vi "Read FOAD.vi"(8 "error in (no error)":errorcluster, 11 "Detector Manager in":refnum<class "Detector Manager.lvclass">=refnum) -> (0 "error out":errorcluster, 2 "Father Of All Detectors.lvclass":refnum<class "Father Of All Detectors.lvclass">, 3 "Detector Manager out":refnum<class "Detector Manager.lvclass">)   [LabVIEW 2026, in "TALOS.lvlib" / "Detector Manager.lvlib" / "Detector Manager.lvclass"]
uses:
  Detector Manager.lvclass
  Classes/Father of all Detectors/Father Of All Detectors.lvclass
  Detector Manager.lvclass/Detector Manager.ctl
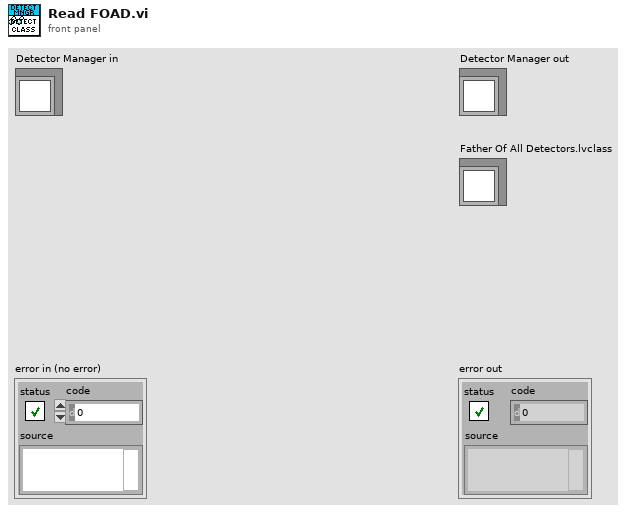
[diagram p1: front panel]
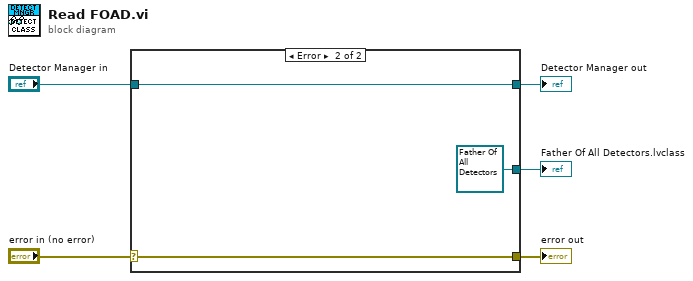
[diagram p0: block diagram]
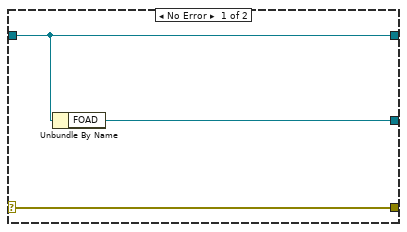
[diagram p2: hidden frame]
diagram:
  n1 = case shown="Error" "error in (no error)" {
    selector: "error in (no error)" -> [w8 w10]
    tunnel: [w8 w10] -> w4
    tunnel: [w7 w11] -> w2
    tunnel: "Detector Manager in" -> [w7 w11]
    tunnel: [w6 refnum<class "Father Of All Detectors.lvclass"> refnum ("FOAD")] -> w1
    frame No Error {
      n2 = Unbundle By Name(w7) -> ("FOAD"=w6:refnum<class "Father Of All Detectors.lvclass">)
    }
    frame Error {
    }
  }
  "error out" <- w4
  "Detector Manager out" <- w2
  "Father Of All Detectors.lvclass" <- w1
